vi "Set Permissions.vi"(8 "error in (no error)":errorcluster, 10 "Remote path":string, 11 "SCP File Transfer in":refnum<class "SCP File Transfer.lvclass">) -> (0 "error out":errorcluster, 3 "SCP File Transfer out":refnum<class "SCP File Transfer.lvclass">)   [LabVIEW 2013, in "PL Framework Configuration Tool.lvlib" / "SCP File Transfer.lvclass"]
uses:
  SCP File Transfer.lvclass
  SCP File Transfer.lvclass/SCP File Transfer.ctl
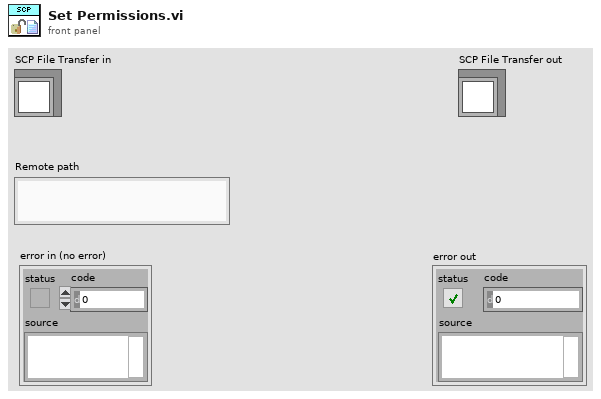
[diagram p1: front panel]
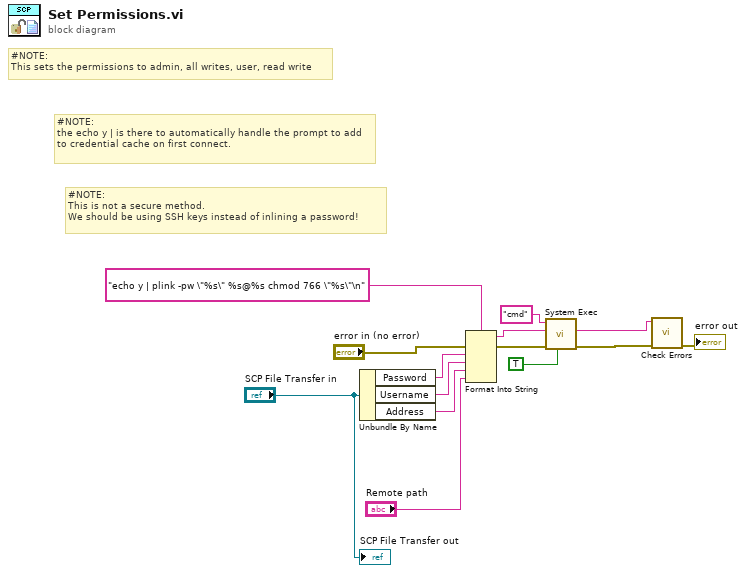
[diagram p0: block diagram]
diagram:
  # "#NOTE:\nThis sets the permissions to admin, all writes, user, read write"
  # "#NOTE:\nthe echo y | is there to automatically handle the prompt to add to credential cache on first connect."
  # "#NOTE:\nThis is not a secure method.\nWe should be using SSH keys instead of inlining a password!"
  n1 = Unbundle By Name("SCP File Transfer in") -> ("Password"=w6:string, "Username"=w5:string, "Address"=w4:string)
  n2 = Format Into String(format string="echo y | plink -pw \"%s\" %s@%s chmod 766 \"%s\"\n", error in="error in (no error)", w6, w5, w4, "Remote path") -> (resulting string=w10:string, error out=w13:errorcluster)  [unwired: 1 in]
  n3 = call <vilib>:"System Exec.vi"("run minimized? (F)"=TRUE, "error in (no error)"=w13, "standard input"=w10, "command line"="cmd") -> ("error out"=w3:errorcluster, "standard error"=w2:string)  [unwired: 4 in, 2 out]
  n4 = call "Check Errors.vi"("error in (no error)"=w3, "standard error"=w2) -> ("error out"=→"error out":errorcluster)  [unwired: 9 in]
  "SCP File Transfer out" <- "SCP File Transfer in"
